vi "TCP_Server.vi"   [LabVIEW 2024]
uses:
  <vilib>/Analysis/NI_AALBase.lvlib
types:
  T1 = enum16{"Standard", "Buffered", "CRLF", "Immediate"}
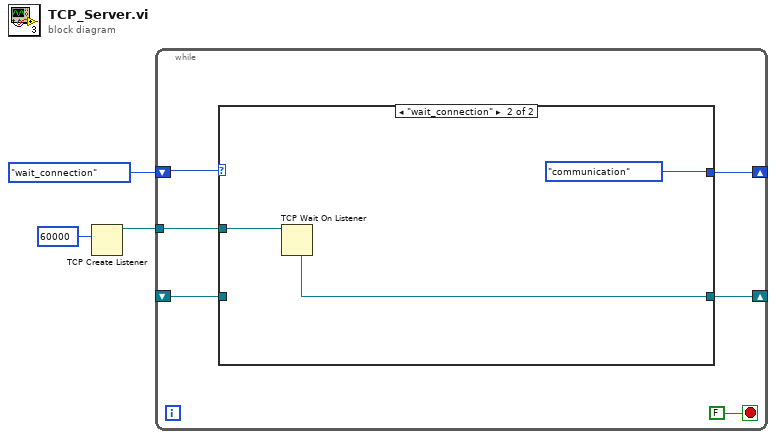
[diagram p0: block diagram]
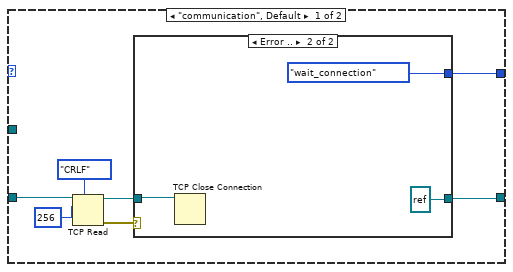
[diagram p2: hidden frame]
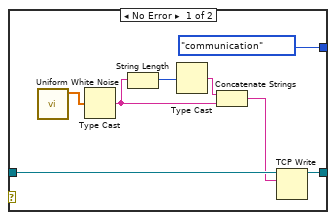
[diagram p3: hidden frame]
diagram:
  n1 = TCP Create Listener(10:u16 60000 ("port")) -> (3:w3:refnum<k5>)  [unwired: 4 in, 2 out]
  n2 = while {
    shift-right: [w6] -> _
    shift-left: enum16{"wait_connection", "communication"}."wait_connection" -> [w4]
    shift-right: [w7] -> _
    shift-left: _ -> [w9]
    tunnel: w3 -> [w8]
    stop <- FALSE stop-if-true
    n3 = case shown="\"wait_connection\"" w4 {
      tunnel: w9 -> [w11 _]
      tunnel: w8 -> [_ w29]
      tunnel: [w12 w28] -> w7
      tunnel: [w13 enum16{"wait_connection", "communication"}."communication"] -> w6
      frame "communication", Default {
        n4 = TCP Read(connection ID=w11, bytes to read=256, 7:T1."CRLF" ("mode (standard)")) -> (connection ID out=w15:refnum<k5>, error out=w10:errorcluster)  [unwired: 2 in, 1 out]
        n5 = case shown="Error .." w10 {
          tunnel: [w24 refnum<k5> refnum ("listener ID")] -> w12
          tunnel: w15 -> [w23 w27]
          tunnel: [enum16{"wait_connection", "communication"}."communication" enum16{"wait_connection", "communication"}."wait_connection"] -> w13
          frame No Error {
            n6 = call <vilib>:"Uniform White Noise.vi"() -> ("uniform white noise"=w22:dbl[])  [unwired: 10 in, 1 out]
            n7 = Type Cast(x=w22) -> (*(type *) &x=w21:string)  [unwired: 1 in]
            n8 = String Length(string=w21) -> (length=w19:i32)
            n9 = Type Cast(x=w19) -> (*(type *) &x=w20:string)  [unwired: 1 in]
            n10 = Concatenate Strings(w20, w21) -> (w18:string)
            n11 = TCP Write(connection ID=w23, data in=w18) -> (connection ID out=w24:refnum<k5>)  [unwired: 2 in, 2 out]
          }
          frame Error {
            n12 = TCP Close Connection(connection ID=w27) -> ()  [unwired: 2 in, 2 out]
          }
        }
      }
      frame "wait_connection" {
        n13 = TCP Wait On Listener(11:w29) -> (4:w28:refnum<k5>)  [unwired: 3 in, 4 out]
      }
    }
  }
